vi "Previous Page.vi"(8 "error in (no error)":errorcluster, 11 "HVAC System Model in":refnum<class "HVAC System Model.lvclass">) -> (0 "error out":errorcluster, 3 "HVAC System Model out":refnum<class "HVAC System Model.lvclass">)   [LabVIEW 2013, in "HVAC System Model.lvlib" / "HVAC System Model.lvclass"]
uses:
  HVAC System Model.lvclass
  HVAC System Model.lvclass/HVAC System Model.ctl
  <vilib>/ActorFrameworkMVC/View Observer/View Registry/View Registry.lvclass/View Registry.ctl
  HVAC System Model Messages/Abstract HVAC System Move In Previous Msg/Abstract HVAC System Move In Previous Msg.lvclass
  <vilib>/ActorFrameworkMVC/View Observer/Data Message/Data Message.lvclass
  <vilib>/ActorFrameworkMVC/View Observer/View Registry/View Registry.lvclass
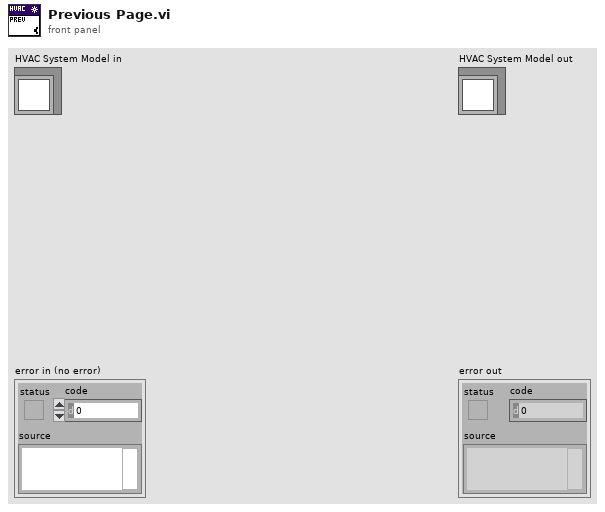
[diagram p1: front panel]
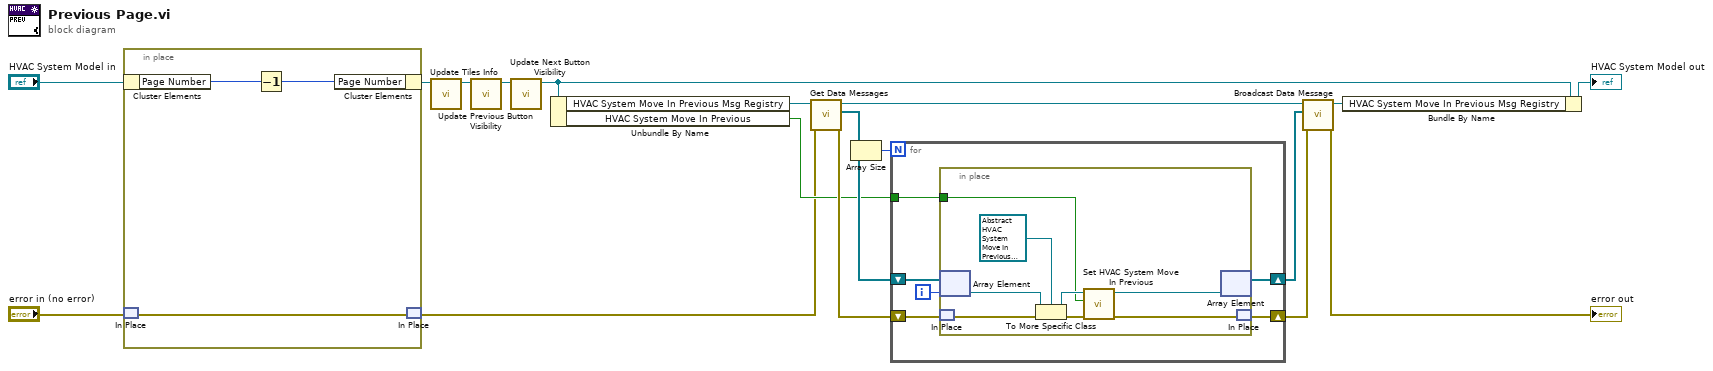
[diagram p0: block diagram]
diagram:
  n1 = in-place {
    n2 = in-place-cluster #1("HVAC System Model in") -> ("Page Number"=w21:i32)
    n3 = in-place-match #2("error in (no error)") -> (w19:errorcluster)
    n4 = Decrement(x=w21) -> (x-1=w20:i32)
    n5 = in-place-cluster #1("Page Number"=w20) -> (w10:refnum<class "HVAC System Model.lvclass">)
    n6 = in-place-match #2(w19) -> (w9:errorcluster)
  }
  n7 = call "Update Tiles Info.vi"("HVAC System Model in"=w10) -> ("HVAC System Model out"=w8:refnum<class "HVAC System Model.lvclass">)  [unwired: 9 in, 1 out]
  n8 = call "Update Previous Button Visibility.vi"("HVAC System Model in"=w8) -> ("HVAC System Model out"=w7:refnum<class "HVAC System Model.lvclass">)  [unwired: 9 in, 1 out]
  n9 = call "Update Next Button Visibility.vi"("HVAC System Model in"=w7) -> ("HVAC System Model out"=w4:refnum<class "HVAC System Model.lvclass">)  [unwired: 9 in, 1 out]
  n10 = Unbundle By Name(w4) -> ("HVAC System Move In Previous Msg Registry"=w18:refnum<class "View Registry.lvclass">, "HVAC System Move In Previous"=w11:bool)
  n11 = call <vilib>:"Get Data Messages.vi"("error in (no error)"=w9, "View Registry in"=w18) -> ("error out"=w14:errorcluster, "Data Messages"=w15:refnum<class "Data Message.lvclass">[], "View Registry out"=w17:refnum<class "View Registry.lvclass">)  [unwired: 7 in]
  n12 = Array Size(array=w15) -> (size(s)=w16:i32)
  n13 = for {
    N: w16 -> [_]
    shift-right: [w26] -> w13
    shift-left: w15 -> [w27]
    shift-right: [w23] -> w12
    shift-left: w14 -> [w25]
    tunnel: w11 -> [w24]
    i -> [w22]
    n14 = in-place {
      in-place-border: w24 -> [w28]
      n15 = in-place-array #3(w27, w22) -> (w33:refnum<class "Data Message.lvclass">)
      n16 = in-place-match #4(w25) -> (w35:errorcluster)
      n17 = To More Specific Class(target class=refnum<class "Abstract HVAC System Move In Previous Msg.lvclass"> refnum ("HVAC System Model.lvlib:Abstract HVAC System Move In Previous Msg.lvclass"), reference=w33, error in=w35) -> (specific class reference=w29:refnum<class "Abstract HVAC System Move In Previous Msg.lvclass">, error out=w32:errorcluster)
      n18 = call "Set HVAC System Move In Previous.vi"("error in (no error)"=w32, "HVAC System Move In Previous"=w28, "Abstract HVAC System Move In Previous Msg in"=w29) -> ("error out"=w31:errorcluster, "Abstract HVAC System Move In Previous Msg out"=w30:refnum<class "Abstract HVAC System Move In Previous Msg.lvclass">)  [unwired: 7 in]
      n19 = in-place-array #3(w30) -> (w26:refnum<class "Data Message.lvclass">[])  [unwired: 1 out]
      n20 = in-place-match #4(w31) -> (w23:errorcluster)
    }
  }
  n21 = call <vilib>:"Broadcast Data Message.vi"("error in (no error)"=w12, "Data Messages"=w13, "View Registry in"=w17) -> ("error out"=→"error out":errorcluster, "View Registry out"=w6:refnum<class "View Registry.lvclass">)  [unwired: 7 in]
  n22 = Bundle By Name(cluster=w4, "HVAC System Move In Previous Msg Registry"=w6) -> (→"HVAC System Model out":refnum<class "HVAC System Model.lvclass">)
